vi "Check Range.vi"(8 "error in (no error)":errorcluster, 10 "max":dbl, 11 "Varian Continuous in":refnum<class "Varian Continuous.lvclass">) -> (0 "error out":errorcluster, 3 "Varian Continuous out":refnum<class "Varian Continuous.lvclass">)   [LabVIEW 2009, in "Varian Continuous.lvclass"]
doc: "Coerce the range to be within this Scanner's physical limits."
uses:
  Varian Continuous.lvclass
  Instruments/Varian Magnet/Varian Max Field.vi
  Instruments/Varian Magnet/Varian Magnet.lvclass
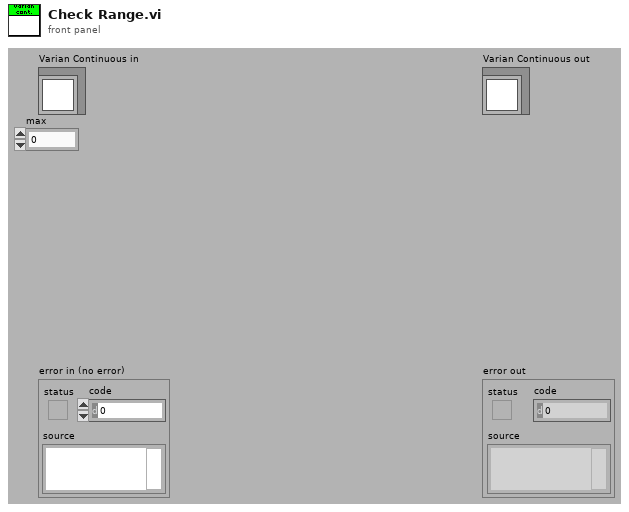
[diagram p1: front panel]
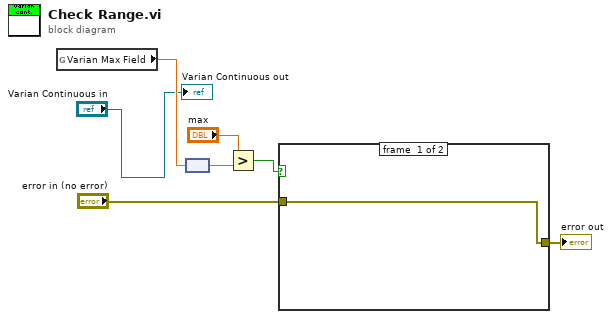
[diagram p0: block diagram]
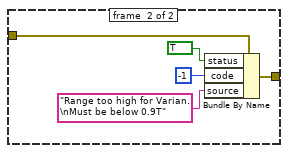
[diagram p2: hidden frame]
diagram:
  n1 = global read "Varian Max Field.vi" "Varian Max Field"() -> (w7:dbl[unit])
  n2 = node(w7) -> (w6:dbl)
  n3 = Greater?(x="max", y=w6) -> (0:w5:bool)
  n4 = case shown="True" w5 {
    tunnel: "error in (no error)" -> [w8 w13]
    tunnel: [w8 w9] -> w4
    frame #0 {
    }
    frame #1 {
      n5 = Bundle By Name(cluster=w13, "status"=TRUE, "code"=-1, "source"="Range too high for Varian.\nMust be below 0.9T") -> (w9:errorcluster)
    }
  }
  "error out" <- w4
  "Varian Continuous out" <- "Varian Continuous in"
